vi "Rewind.vi"(8 "Error In":errorcluster, 11 "ByteBuffer In":refnum<class "ByteBuffer.lvclass">) -> (0 "Error Out":errorcluster, 3 "ByteBuffer Out":refnum<class "ByteBuffer.lvclass">)   [LabVIEW 2015, in "ByteBuffer.lvclass"]
doc: "Clears this buffer, the position is set to zero, the limit is set to the capacity, and the mark is discarded."
uses:
  ByteBuffer.lvclass
  properties/position/Set Position.vi
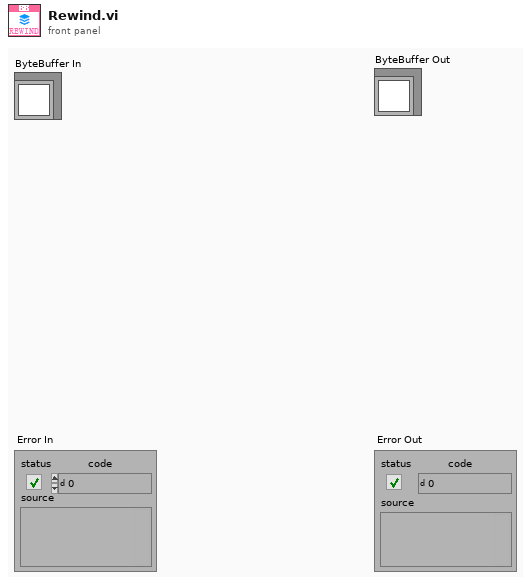
[diagram p1: front panel]
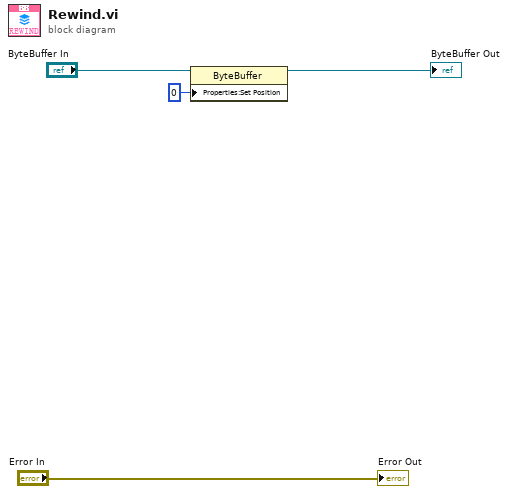
[diagram p0: block diagram]
diagram:
  n1 = property class="ByteBuffer"(reference="ByteBuffer In", "Properties:Set Position"=u32 0 ("Set Position")) -> (reference out=→"ByteBuffer Out":refnum<class "ByteBuffer.lvclass">)  [unwired: 1 in, 1 out]
  "Error Out" <- "Error In"
